vi "test-PID-testSetSetpoint.vi"() -> (3 "All Passed":bool)   [LabVIEW 2019]
uses:
  <vilib>/Rock Robotics/WPI/ThirdParty/JAS_Junk/TrajLib/PID_CONTROLLER.ctl
  <vilib>/Rock Robotics/WPI/ThirdParty/JAS_Junk/TrajLib/PIDController_NewPeriod.vi
  <vilib>/Rock Robotics/WPI/ThirdParty/JAS_Junk/TrajLib/PIDController_SetSetpoint.vi
  <vilib>/Rock Robotics/WPI/ThirdParty/JAS_Junk/TrajLib/PIDController_Calculate_PV.vi
  <vilib>/Rock Robotics/SystemInterfaces/NetworkCommunication/NetComm_UsageReport_report.vi
  <vilib>/Rock Robotics/WPI/ThirdParty/JAS_Junk/TrajLib/ControllerUtil_GetModulusError.vi
  <vilib>/Rock Robotics/WPI/ThirdParty/JAS_Junk/TrajLib/Util_LibraryGlobals.vi
  <vilib>/Rock Robotics/WPI/ThirdParty/JAS_Junk/TrajLib/Trajectory_Library.lvlib
panel:
  out "T3 Passed":bool
  out "T2 Passed":bool
  out "T1 Passed":bool
  out "T0 Passed":bool
  out "T0 PID CTRL":T1={"Kp"=0.0, "Ki"=0.0, "Kd"=0.0, "Period"=0.0, "Max_Integral"=0.0, "Min_Integral"=0.0, "Max_Input"=0.0, "Min_Input"=0.0, "Continuous"=FALSE, "PositionError"=0.0, "VelocityError"=0.0, "PrevError"=0.0, "TotalError"=0.0, "PositionTolerance"=0.0, "VelocityTolerance"=0.0, "SetPoint"=0.0, "Kf"=0.0, "Prev_Deriv"=0.0, "Prev_Deriv 2"=0.0, "DerivativeFilter"=FALSE, "Min_Output"=-9.99e+35, "Max_Output"=9.9e+35, "Prev_F_P"=0.0, "Prev_F_P_2"=0.0, "AntiWindupActive"=FALSE, "Measurement"=0.0} {"Measurement" format="%16_6e"; "Prev_F_P_2" format="%16_6e"; "Prev_F_P" format="%16_6e"; "Max_Output" format="%16_6e"; "Min_Output" format="%16_6e"; "Prev_Deriv 2" format="%16_6e"; "Prev_Deriv" format="%16_6e"; "Kf" format="%16_6e"; "SetPoint" format="%16_6e"; "VelocityTolerance" format="%16_6e"; "PositionTolerance" format="%16_6e"; "TotalError" format="%16_6e"; "PrevError" format="%16_6e"; "VelocityError" format="%16_6e"; "PositionError" format="%16_6e"; "Min_Input" format="%16_6e"; "Max_Input" format="%16_6e"; "Min_Integral" format="%16_6e"; "Max_Integral" format="%16_6e"; "Period" format="%16_6e"; "Kd" format="%16_6e"; "Ki" format="%16_6e"; "Kp" format="%16_6e"}
  out "T3 -- Output =":dbl
  out "T2 -- Output  = -0.01":dbl
  out "T1 -- Output  = -0.1":dbl
  out "T0 -- Output < 0":dbl
  # "PID TEST"
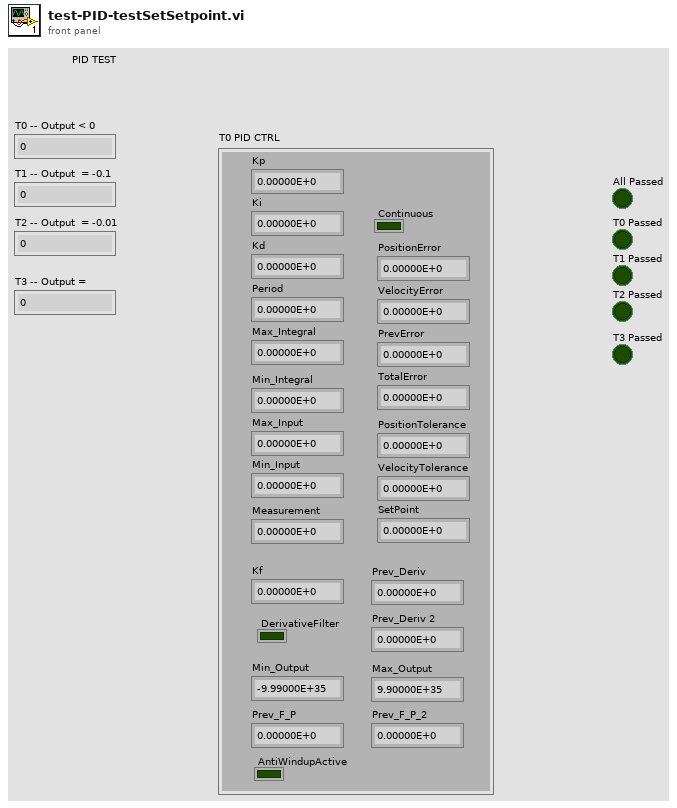
[diagram p1: front panel]
types:
  T1 = typedef "Trajectory_Library.lvlib/PID_CONTROLLER.ctl" = cluster{"Kp":dbl, "Ki":dbl, "Kd":dbl, "Period":dbl, "Max_Integral":dbl, "Min_Integral":dbl, "Max_Input":dbl, "Min_Input":dbl, "Continuous":bool, "PositionError":dbl, "VelocityError":dbl, "PrevError":dbl, "TotalError":dbl, "PositionTolerance":dbl, "VelocityTolerance":dbl, "SetPoint":dbl, "Kf":dbl, "Prev_Deriv":dbl, "Prev_Deriv 2":dbl, "DerivativeFilter":bool, "Min_Output":dbl, "Max_Output":dbl, "Prev_F_P":dbl, "Prev_F_P_2":dbl, "AntiWindupActive":bool, "Measurement":dbl}
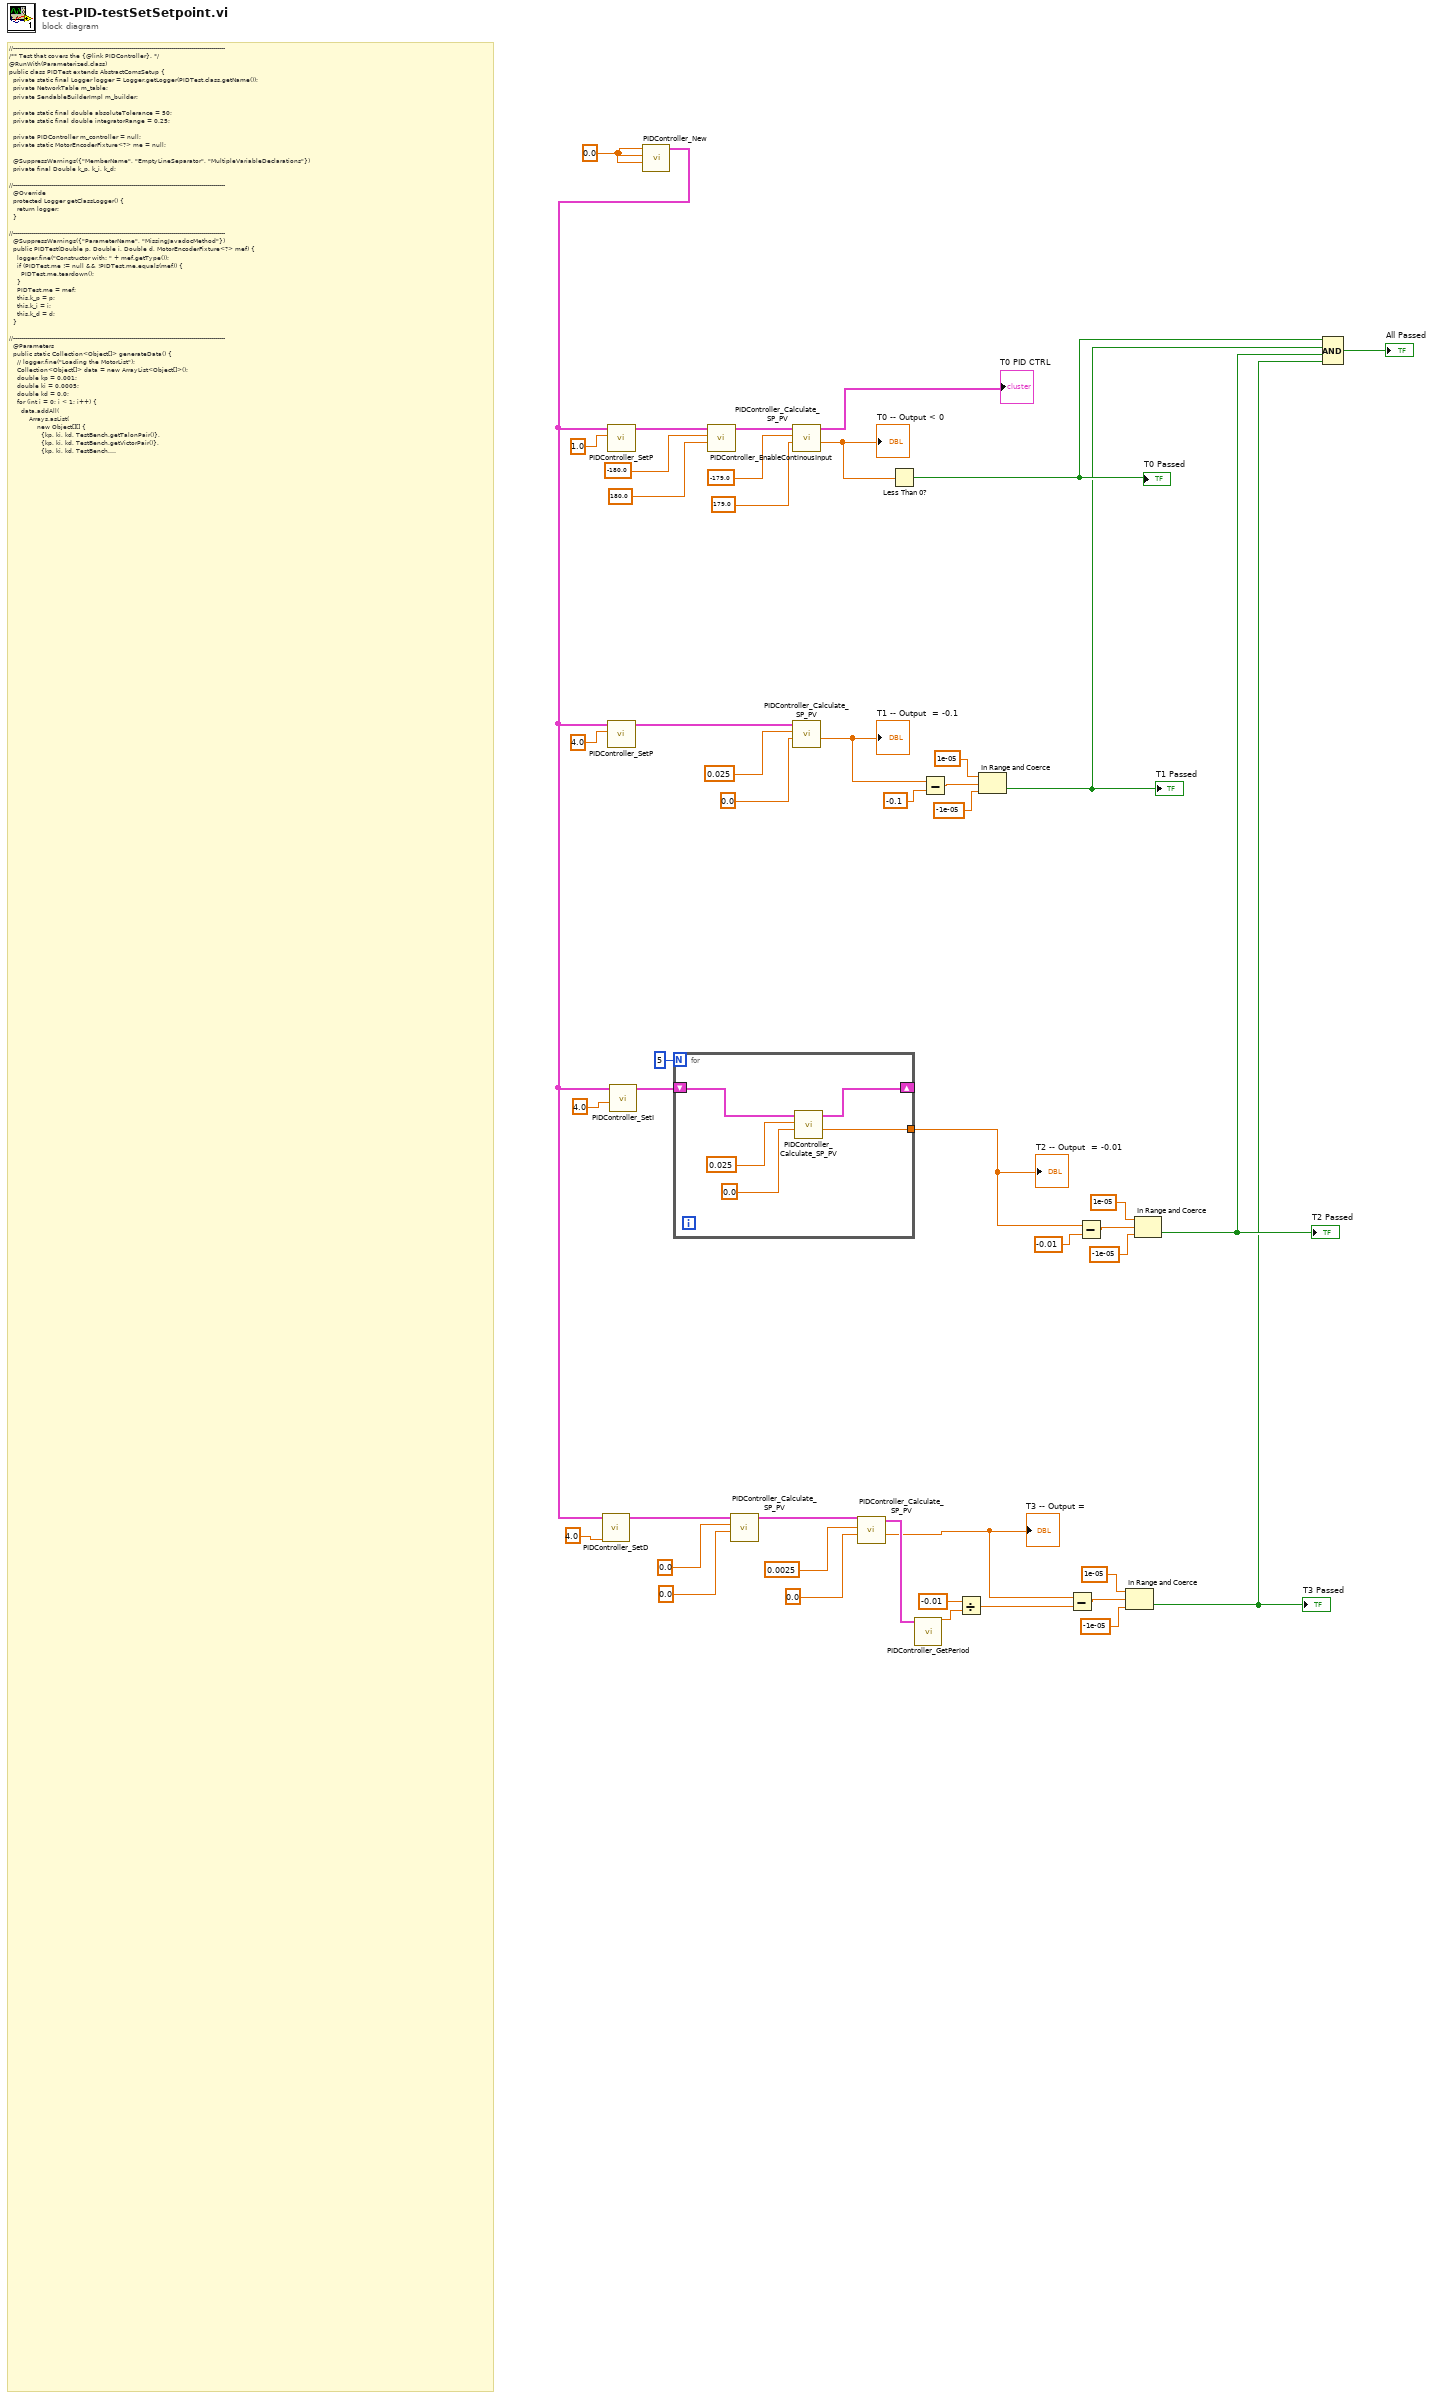
[diagram p0: block diagram]
diagram:
  w48 = 0.0 ("Kp")
  # "//----------------------------------------------------------------------------------------------------------\n/** Test that covers the {@link PIDController}. */\n@RunWith(Parameterized.class)\npublic class PIDTest extends AbstractComsSetup {\n  private static final Logger logger = Logger.getLogger(PIDTest.class.getName());\n  private NetworkTable m_table;\n  private SendableBuilderImpl m_builder;\n\n  private static final double absoluteTolerance = 50;\n  private static final double integratorRange = 0.25;\n\n  private PIDController m_controller = null;\n  private static MotorEncoderFixture<?> me = null;\n\n  @SuppressWarnings({\"MemberName\", \"EmptyLineSeparator\", \"MultipleVariableDeclarations\"})\n  private final Double k_p, k_i, k_d;\n\n//----------------------------------------------------------------------------------------------------------\n  @Override\n  protected Logger getClassLogger() {\n    return logger;\n  }\n\n//----------------------------------------------------------------------------------------------------------\n  @SuppressWarnings({\"ParameterName\", \"MissingJavadocMethod\"})\n  public PIDTest(Double p, Double i, Double d, MotorEncoderFixture<?> mef) {\n    logger.fine(\"Constructor with: \" + mef.getType());\n    if (PIDTest.me != null && !PIDTest.me.equals(mef)) {\n      PIDTest.me.teardown();\n    }\n    PIDTest.me = mef;\n    this.k_p = p;\n    this.k_i = i;\n    this.k_d = d;\n  }\n\n//----------------------------------------------------------------------------------------------------------\n  @Parameters\n  public static Collection<Object[]> generateData() {\n    // logger.fine(\"Loading the MotorList\");\n    Collection<Object[]> data = new ArrayList<Object[]>();\n    double kp = 0.001;\n    double ki = 0.0005;\n    double kd = 0.0;\n    for (int i = 0; i < 1; i++) {\n      data.addAll(\n          Arrays.asList(\n              new Object[][] {\n                {kp, ki, kd, TestBench.getTalonPair()},\n                {kp, ki, kd, TestBench.getVictorPair()},\n                {kp, ki, kd, TestBench.getJaguarPair()}\n              }));\n    }\n    return data;\n  }\n\n//----------------------------------------------------------------------------------------------------------\n  @BeforeClass\n  public static void setUpBeforeClass() {}\n\n//----------------------------------------------------------------------------------------------------------\n  @AfterClass\n  public static void tearDownAfterClass() {\n    logger.fine(\"TearDownAfterClass: \" + me.getType());\n    me.teardown();\n    me = null;\n  }\n\n//----------------------------------------------------------------------------------------------------------\n  @Before\n  public void setUp() {\n    logger.fine(\"Setup: \" + me.getType());\n    me.setup();\n    m_table = NetworkTableInstance.getDefault().getTable(\"TEST_PID\");\n    m_builder = new SendableBuilderImpl();\n    m_builder.setTable(m_table);\n    m_controller = new PIDController(k_p, k_i, k_d);\n    m_controller.initSendable(m_builder);\n  }\n\n//----------------------------------------------------------------------------------------------------------\n  @After\n  public void tearDown() {\n    logger.fine(\"Teardown: \" + me.getType());\n    m_controller = null;\n    me.reset();\n  }\n\n//----------------------------------------------------------------------------------------------------------\n  private void setupTolerance() {\n    m_controller.setTolerance(absoluteTolerance);\n  }\n\n//----------------------------------------------------------------------------------------------------------\n  private void setupIntegratorRange() {\n    m_controller.setIntegratorRange(-integratorRange, integratorRange);\n  }\n\n//----------------------------------------------------------------------------------------------------------\n  @Test\n  public void testInitialSettings() {\n    setupTolerance();\n    setupIntegratorRange();\n    double reference = 2500.0;\n    m_controller.setSetpoint(reference);\n    assertEquals(\n        \"PID.getPositionError() did not start at \" + reference,\n        reference,\n        m_controller.getPositionError(),\n        0);\n    m_builder.update();\n    assertEquals(k_p, m_table.getEntry(\"Kp\").getDouble(9999999), 0);\n    assertEquals(k_i, m_table.getEntry(\"Ki\").getDouble(9999999), 0);\n    assertEquals(k_d, m_table.getEntry(\"Kd\").getDouble(9999999), 0);\n    assertEquals(reference, m_table.getEntry(\"reference\").getDouble(9999999), 0);\n    assertFalse(m_table.getEntry(\"enabled\").getBoolean(true));\n  }\n\n//----------------------------------------------------------------------------------------------------------\n  @Test\n  public void testSetSetpoint() {\n    setupTolerance();\n    setupIntegratorRange();\n    double reference = 2500.0;\n    m_controller.setSetpoint(reference);\n    assertEquals(\"Did not correctly set reference\", reference, m_controller.getSetpoint(), 1e-3);\n  }\n\n//----------------------------------------------------------------------------------------------------------\n  @Test(timeout = 10000)\n  public void testRotateToTarget() {\n    setupTolerance();\n    setupIntegratorRange();\n    double reference = 1000.0;\n    assertEquals(pidData() + \"did not start at 0\", 0, me.getMotor().get(), 0);\n    m_controller.setSetpoint(reference);\n    assertEquals(\n        pidData() + \"did not have an error of \" + reference,\n        reference,\n        m_controller.getPositionError(),\n        0);\n    Notifier pidRunner =\n        new Notifier(\n            () -> me.getMotor().set(m_controller.calculate(me.getEncoder().getDistance())));\n    pidRunner.startPeriodic(m_controller.getPeriod());\n    Timer.delay(5);\n    pidRunner.stop();\n    assertTrue(\n        pidData() + \"Was not on Target. Controller Error: \" + m_controller.getPositionError(),\n        m_controller.atSetpoint());\n\n    pidRunner.close();\n  }\n\n//----------------------------------------------------------------------------------------------------------\n  private String pidData() {\n    return me.getType()\n        + \" PID {P:\"\n        + m_controller.getP()\n        + \" I:\"\n        + m_controller.getI()\n        + \" D:\"\n        + m_controller.getD()\n        + \"} \";\n  }\n\n//----------------------------------------------------------------------------------------------------------\n  @Test(expected = RuntimeException.class)\n  public void testOnTargetNoToleranceSet() {\n    setupIntegratorRange();\n    assertFalse(m_controller.atSetpoint());\n  }\n}"
  n1 = call <vilib>:"PIDController_New.vi"("Kd"=w48, "Ki"=w48, "Kp"=w48) -> ("PID_CONTROLLER"=w29:T1)  [unwired: 8 in]
  n2 = call <vilib>:"PIDController_SetD.vi"("Kd"=4.0 ("Kp"), "in PID_CONTROLLER"=w29) -> ("out PID_CONTROLLER"=w32:T1)  [unwired: 9 in]
  n3 = call <vilib>:"PIDController_SetP.vi"("Kp"=1.0, "in PID_CONTROLLER"=w29) -> ("out PID_CONTROLLER"=w46:T1)  [unwired: 9 in]
  n4 = call <vilib>:"PIDController_SetP.vi"("Kp"=4.0, "in PID_CONTROLLER"=w29) -> ("out PID_CONTROLLER"=w37:T1)  [unwired: 9 in]
  n5 = call <vilib>:"PIDController_SetI.vi"("Ki"=4.0 ("Kp"), "in PID_CONTROLLER"=w29) -> ("out PID_CONTROLLER"=w35:T1)  [unwired: 9 in]
  n6 = for {
    N: 5 -> [_]
    tunnel: [w51] -> w14
    shift-right: [w49] -> _
    shift-left: w35 -> [w50]
    n7 = call <vilib>:"PIDController_Calculate_SP_PV.vi"("SP-SetPoint"=0.0, "PV-Measurement"=0.025, "in PID_CONTROLLER"=w50) -> ("CO-ControlOutput"=w51:dbl, "out PID_CONTROLLER"=w49:T1)  [unwired: 7 in]
  }
  "T2 -- Output  = -0.01" <- w14
  n8 = call <vilib>:"PIDController_EnableContinousInput.vi"("MaxInput"=180.0, "MinInput"=-180.0, "in PID_CONTROLLER"=w46) -> ("out PID_CONTROLLER"=w43:T1)  [unwired: 8 in]
  n9 = call <vilib>:"PIDController_Calculate_SP_PV.vi"("SP-SetPoint"=0.0, "PV-Measurement"=0.0, "in PID_CONTROLLER"=w32) -> ("out PID_CONTROLLER"=w26:T1)  [unwired: 7 in, 1 out]
  n10 = call <vilib>:"PIDController_Calculate_SP_PV.vi"("SP-SetPoint"=179.0, "PV-Measurement"=-179.0, "in PID_CONTROLLER"=w43) -> ("CO-ControlOutput"=w24:dbl, "out PID_CONTROLLER"=→"T0 PID CTRL":T1)  [unwired: 7 in]
  "T0 -- Output < 0" <- w24
  n11 = call <vilib>:"PIDController_Calculate_SP_PV.vi"("SP-SetPoint"=0.0, "PV-Measurement"=0.025, "in PID_CONTROLLER"=w37) -> ("CO-ControlOutput"=w22:dbl)  [unwired: 7 in, 1 out]
  "T1 -- Output  = -0.1" <- w22
  n12 = call <vilib>:"PIDController_Calculate_SP_PV.vi"("SP-SetPoint"=0.0, "PV-Measurement"=0.0025, "in PID_CONTROLLER"=w26) -> ("CO-ControlOutput"=w6:dbl, "out PID_CONTROLLER"=w13:T1)  [unwired: 7 in]
  "T3 -- Output =" <- w6
  n13 = Less Than 0?(x=w24) -> (x < 0?=w5:bool)
  "T0 Passed" <- w5
  n14 = call <vilib>:"PIDController_GetPeriod.vi"("in PID_CONTROLLER"=w13) -> ("Period"=w12:dbl)  [unwired: 10 in]
  n15 = Subtract(x=w22, y=-0.1) -> (x-y=w19:dbl)
  n16 = Divide(x=-0.01, y=w12) -> (x/y=w7:dbl)
  n17 = In Range and Coerce(upper limit=1e-05, x=w19, lower limit=-1e-05 ("upper limit")) -> (In Range?=w4:bool)  [unwired: 1 out]
  "T1 Passed" <- w4
  n18 = Subtract(x=w6, y=w7) -> (x-y=w9:dbl)
  n19 = Subtract(x=w14, y=-0.01) -> (x-y=w16:dbl)
  n20 = In Range and Coerce(upper limit=1e-05, x=w9, lower limit=-1e-05 ("upper limit")) -> (In Range?=w1:bool)  [unwired: 1 out]
  "T3 Passed" <- w1
  n21 = In Range and Coerce(upper limit=1e-05, x=w16, lower limit=-1e-05 ("upper limit")) -> (In Range?=w2:bool)  [unwired: 1 out]
  "T2 Passed" <- w2
  n22 = Compound Arithmetic op=AND(w5, w4, w2, w1) -> (→"All Passed":bool)
